vi "gestosc_prawdop.vi"() -> ()   [LabVIEW 2025]
panel:
  out "gestosc prawd":cluster{dbl[], dbl[]}(graph)
  in  "liczba cykli":i64
  in  "Sygnal":T1(ring)
  in  "phase":dbl
  in  "Amp":dbl
  in  "samples":i32=128
  in  "rozdzielczosc":dbl
  out "histogram":cluster{dbl[], i32[]}(graph)
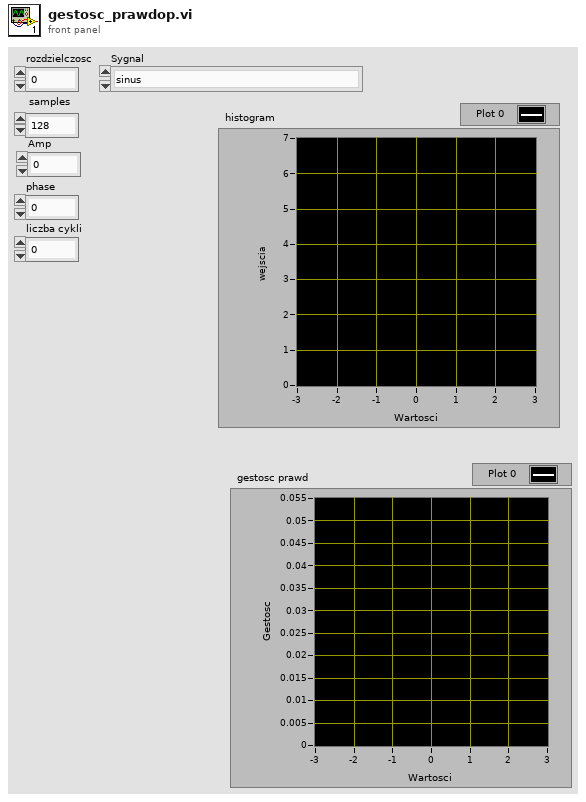
[diagram p1: front panel]
types:
  T1 = enum16{"sinus", "prostokat", "pila", "trojkat", "rozklad losowy", "rozklad normalny"}
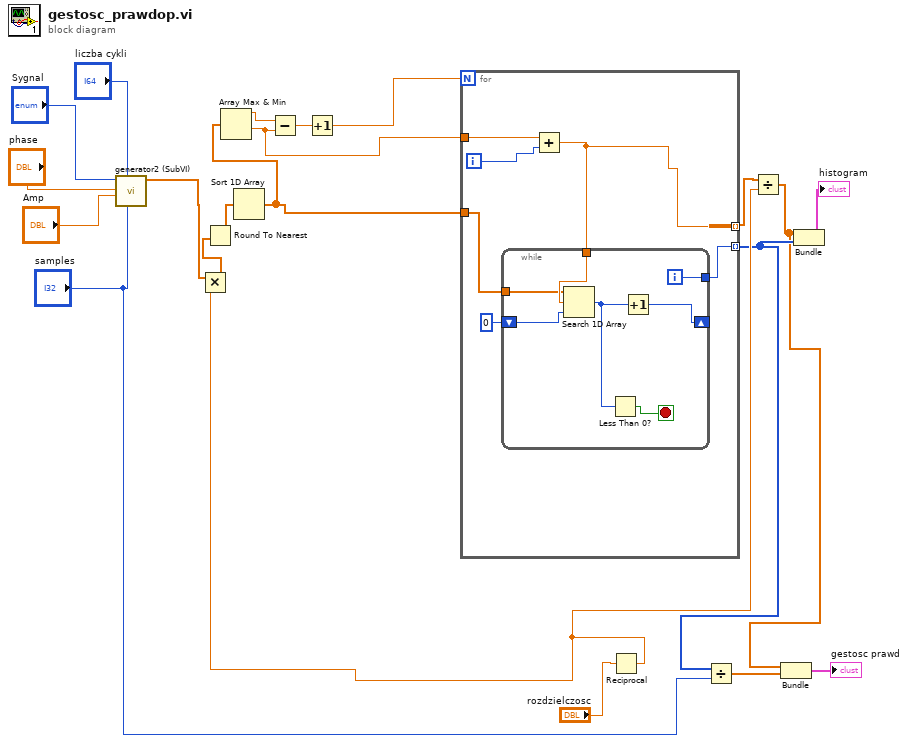
[diagram p0: block diagram]
diagram:
  n1 = call "generator2 (SubVI).vi"("samples"="samples", "liczba cykli"="liczba cykli", "Amp"="Amp", "phase"="phase", "Sygnal"="Sygnal") -> ("Gaussian noise pattern"=w10:dbl[])  [unwired: 6 in]
  n2 = Reciprocal(x="rozdzielczosc") -> (1/x=w11:dbl)
  n3 = Multiply(x=w10, y=w11) -> (x*y=w14:dbl[])
  n4 = Round To Nearest(number=w14) -> (nearest integer value=w13:dbl[])
  n5 = Sort 1D Array(array=w13) -> (sorted array=w17:dbl[])
  n6 = Array Max & Min(array=w17) -> (max value=w19:dbl, min value=w18:dbl)  [unwired: 2 out]
  n7 = Subtract(x=w19, y=w18) -> (x-y=w21:dbl)
  n8 = Increment(x=w21) -> (x+1=w20:dbl)
  n9 = for {
    N: w20 -> [_]
    tunnel: w18 -> [w27]
    tunnel: w17 -> [w26]
    tunnel: [w25] -> w4 mode=indexing
    tunnel: [w24] -> w15 mode=indexing
    i -> [w22]
    n10 = Add(x=w27, y=w22) -> (x+y=w24:dbl)
    n11 = while {
      tunnel: w24 -> [w33]
      tunnel: w26 -> [w32]
      shift-right: [w30] -> _
      shift-left: 0 -> [w31]
      tunnel: [w28] -> w25
      i -> [w28]
      stop <- w34 stop-if-true
      n12 = Search 1D Array(1D array=w32, element=w33, start index (0)=w31) -> (index of element=w29:i32)
      n13 = Less Than 0?(x=w29) -> (x < 0?=w34:bool)
      n14 = Increment(x=w29) -> (x+1=w30:i32)
    }
  }
  n15 = Divide(x=w4, y="samples") -> (x/y=w2:dbl[])
  n16 = Divide(x=w15, y=w11) -> (x/y=w3:dbl[])
  n17 = Bundle(w3, w2) -> (→"gestosc prawd":cluster{dbl[], dbl[]})  [unwired: 1 in]
  n18 = Bundle(w3, w4) -> (→"histogram":cluster{dbl[], i32[]})  [unwired: 1 in]
